vi "Python@SetCaptureFile(Worker)__Parameter.vi"(1 "ParamterIn":string) -> (0 "ParamterOut":string)   [LabVIEW 2020]
uses:
  MainFrame/Global.vi
panel:
  in  "Session":string(combo)
  out "Image":T1(plugin-control)
  in  "Picture":string(combo)
  in  "PythonName":string(combo)
  in  "CamName":string(combo)
  in  "Confirm":bool
  # "Python@SetCaptureFile(worker) $Worker,$Capture,$Picture,$PythonName"
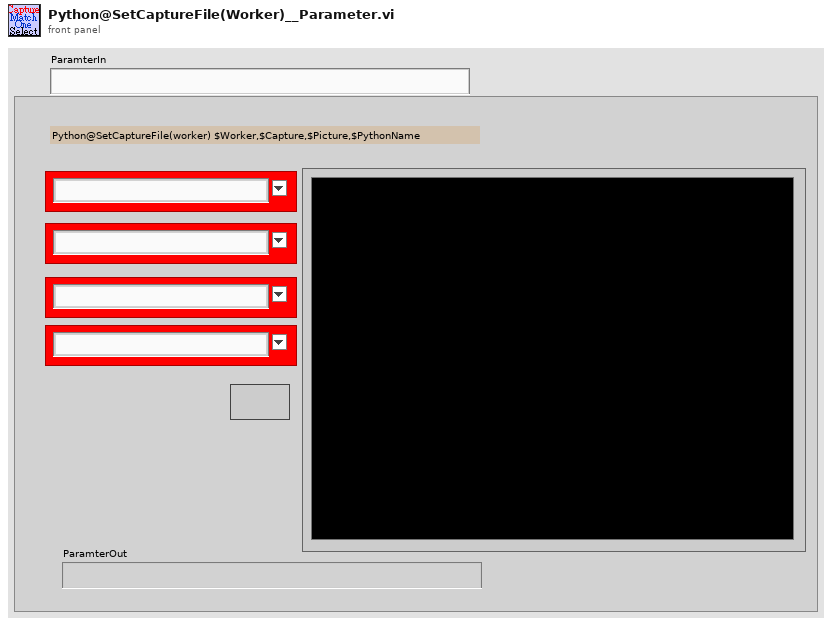
[diagram p1: front panel]
types:
  T1 = typedef "IMAQ Image.ctl" = refnum<image>
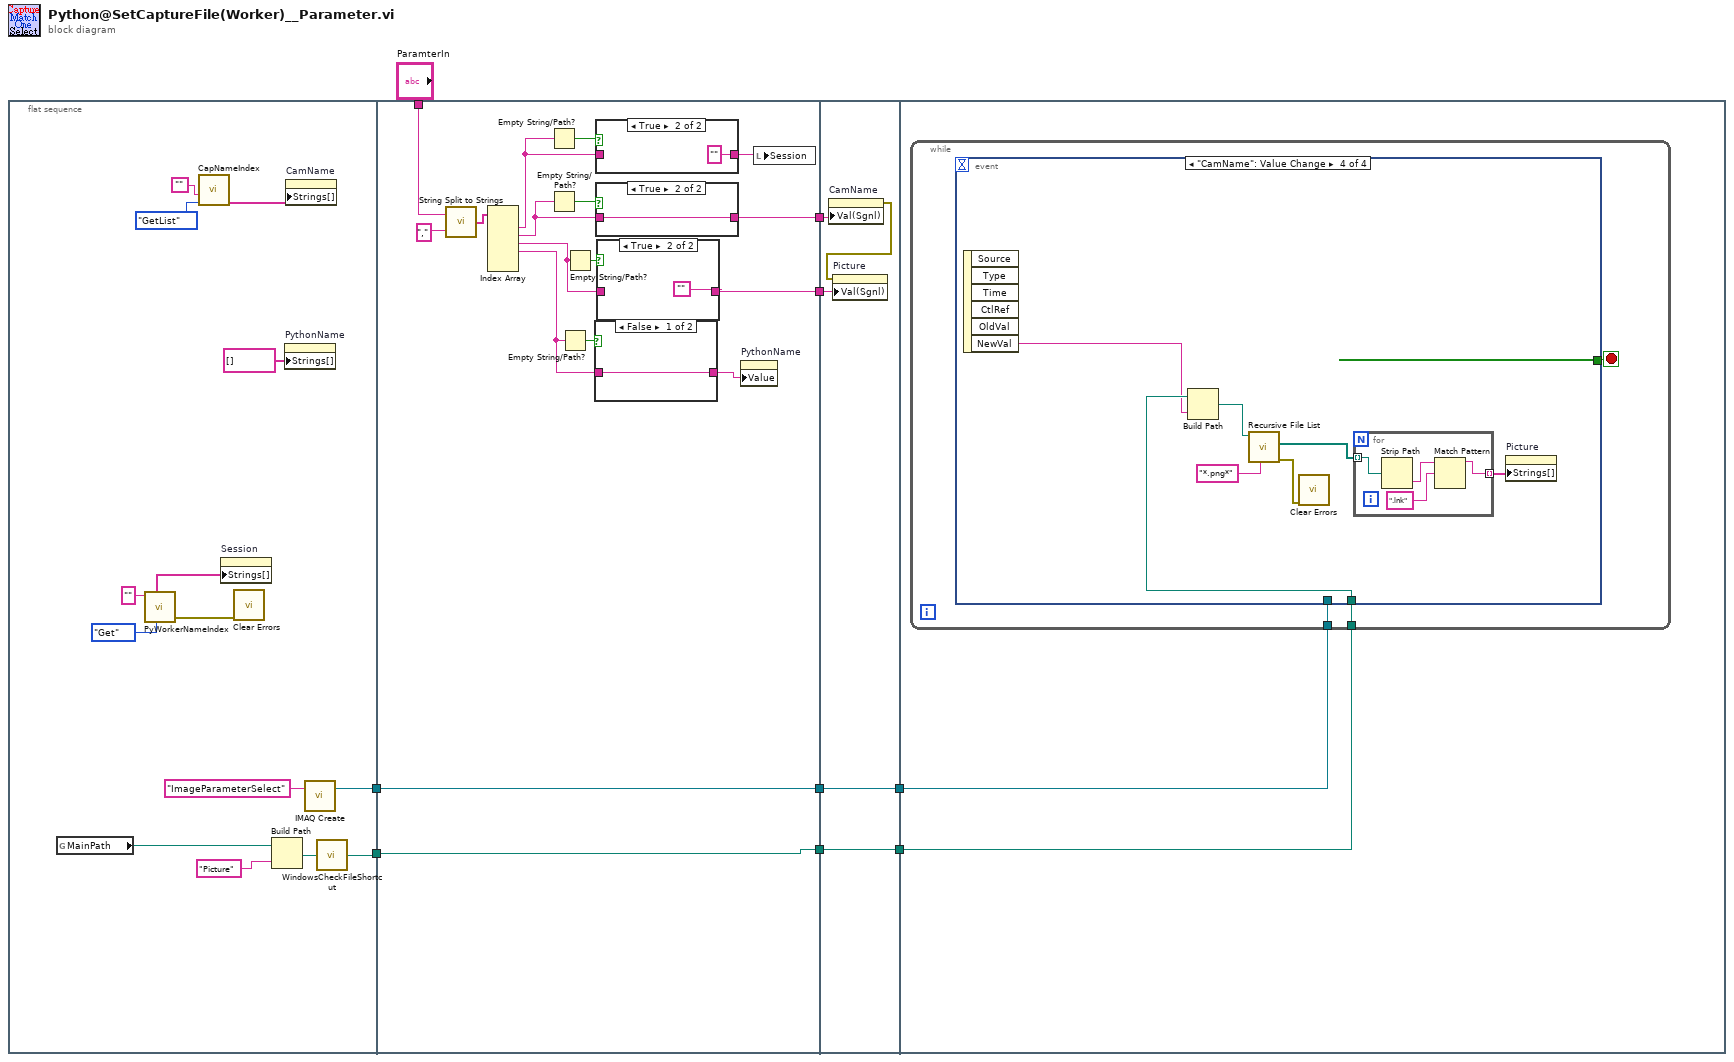
[diagram p0: block diagram]
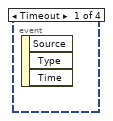
[diagram p6: hidden frame]
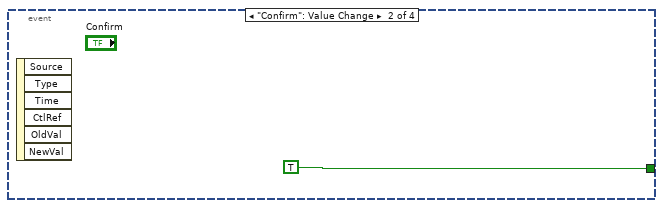
[diagram p7: hidden frame]
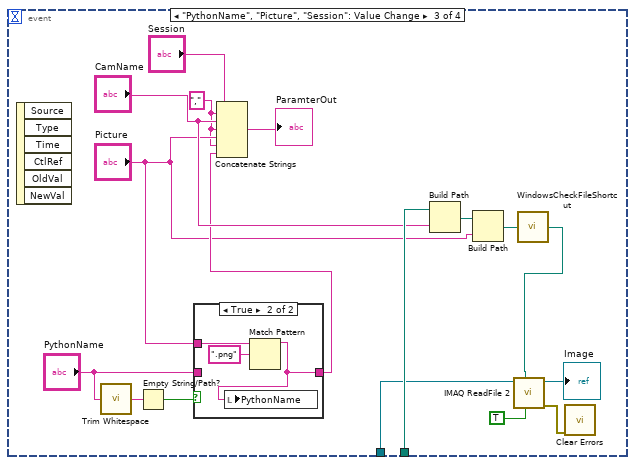
[diagram p8: hidden frame]
diagram:
  n1 = flat-sequence {
    tunnel: [w19] -> w8
    tunnel: [w10] -> w3
    tunnel: "ParamterIn" -> [w38]
    tunnel: w8 -> [w31]
    tunnel: [w31] -> w7
    tunnel: [w29] -> w4
    tunnel: w3 -> [w29]
    tunnel: [w28] -> w2
    tunnel: [w27] -> w1
    tunnel: w7 -> [w53]
    tunnel: [w53] -> w6
    tunnel: [w52] -> w5
    tunnel: w4 -> [w52]
    tunnel: w2 -> [w51]
    tunnel: w1 -> [w49]
    tunnel: w6 -> [w55]
    tunnel: w5 -> [w54]
    frame #0 {
      n2 = global read "Global.vi" "MainPath"() -> (w17:path)
      n3 = call "PyWorkerNameIndex.vi"("OP"=enum16{"Init", "Get", "Set"}."Get", "WrokerName"="" ("SessionIn")) -> ("error out"=w12:errorcluster, "PythonWorkerNameS"=w13:string[])  [unwired: 6 in, 2 out]
      n4 = call "CapNameIndex.vi"("OP"=enum16{"AddCam", "GetIndex", "Init", "GetList"}."GetList", "CamName"="") -> ("DeviceList"=w22:string[])  [unwired: 2 in, 3 out]
      n5 = property on="Session" class="CmbBox"("Strings[]"=w13) -> ()  [unwired: 2 in, 2 out]
      n6 = call <vilib>:"Clear Errors.vi"("error in (no error)"=w12) -> ()  [unwired: 5 in, 2 out]
      n7 = Build Path(base path=w17, name or relative path="Picture") -> (appended path=w11:path)
      n8 = property on="PythonName" class="CmbBox"("Strings[]"=string[] [] ("Strings []")) -> ()  [unwired: 2 in, 2 out]
      n9 = property on="CamName" class="CmbBox"("Strings[]"=w22) -> ()  [unwired: 2 in, 2 out]
      n10 = call "IMAQ Create"("Image Name"="ImageParameterSelect") -> ("New Image"=w19:T1)  [unwired: 4 in, 1 out]
      n11 = call "WindowsCheckFileShortcut.vi"("LinkPath"=w11) -> ("TargetPath"=w10:path)  [unwired: 4 in]
    }
    frame #1 {
      n12 = call "String Split to Strings.vi"("search string/char (-)"=",", "String"=w38) -> ("Array"=w40:string[])
      n13 = Index Array(array=w40) -> (element #1=w25:string, element #2=w30:string, element #3=w32:string, element #4=w35:string)  [unwired: 6 in, 2 out]
      n14 = Empty String/Path?(string/path=w25) -> (empty?=w26:bool)
      n15 = Empty String/Path?(string/path=w30) -> (empty?=w37:bool)
      n16 = Empty String/Path?(string/path=w35) -> (empty?=w36:bool)
      n17 = Empty String/Path?(string/path=w32) -> (empty?=w33:bool)
      n18 = case shown="False" w36 {
        tunnel: [w45 w46] -> w34
        tunnel: w35 -> [w45 w46]
        frame False {
        }
        frame True {
        }
      }
      n19 = case shown="True" w26 {
        tunnel: w25 -> [w41 _]
        tunnel: [w41 ""] -> w24
        frame False {
        }
        frame True {
        }
      }
      n20 = case shown="True" w37 {
        tunnel: w30 -> [w47 w48]
        tunnel: [w47 w48] -> w27
        frame False {
        }
        frame True {
        }
      }
      n21 = case shown="True" w33 {
        tunnel: [w43 ""] -> w28
        tunnel: w32 -> [w43 _]
        frame False {
        }
        frame True {
        }
      }
      n22 = property on="PythonName" class="CmbBox"("Value"=w34) -> ()  [unwired: 2 in, 2 out]
      n23 = local write "Session"(w24) -> ()
    }
    frame #2 {
      n24 = property on="CamName" class="CmbBox"("Val(Sgnl)"=w49) -> (error out=w50:errorcluster)  [unwired: 2 in, 1 out]
      n25 = property on="Picture" class="CmbBox"(error in=w50, "Val(Sgnl)"=w51) -> ()  [unwired: 1 in, 2 out]
    }
    frame #3 {
      n26 = while {
        tunnel: w55 -> [w57]
        tunnel: w54 -> [w56]
        stop <- w58 stop-if-true
        n27 = event shown="[3] \"CamName\": Value Change" {
          selector: _ -> [_ _ _ _]
          dyn-events: _ -> [_ _ _ _]
          timeout: _ -> [_ _ _ _]
          tunnel: [_ TRUE _ _] -> w58
          tunnel: w57 -> [_ _ w65 _]
          tunnel: w56 -> [_ _ w75 w84]
          event Timeout {
            n28 = event-data() -> ()  [unwired: 1 in, 3 out]
          }
          event "Confirm": Value Change {
            n29 = event-data() -> ()  [unwired: 1 in, 6 out]
          }
          event "PythonName", "Picture", "Session": Value Change {
            w63 = "," ("string")
            n30 = event-data() -> ()  [unwired: 1 in, 6 out]
            n31 = call <vilib>:"Trim Whitespace.vi"("string"="PythonName") -> ("trimmed string"=w70:string)  [unwired: 1 in]
            n32 = Empty String/Path?(string/path=w70) -> (empty?=w69:bool)
            n33 = case shown="True" w69 {
              tunnel: "PythonName" -> [w77 _]
              tunnel: [w77 w78] -> w67
              tunnel: "Picture" -> [_ w80]
              frame False {
              }
              frame True {
                n34 = Match Pattern(string=w80, regular expression=".png") -> (before substring=w78:string)  [unwired: 1 in, 3 out]
                n35 = local write "PythonName"(w78) -> ()
              }
            }
            n36 = Concatenate Strings("Session", w63, "CamName", w63, "Picture", w63, w67) -> (→"ParamterOut":string)
            n37 = Build Path(base path=w75, name or relative path="CamName") -> (appended path=w73:path)
            n38 = Build Path(base path=w73, name or relative path="Picture") -> (appended path=w61:path)
            n39 = call "WindowsCheckFileShortcut.vi"("LinkPath"=w61) -> ("TargetPath"=w60:path)  [unwired: 4 in]
            n40 = call "IMAQ ReadFile 2"("Use File Path Image Type"=TRUE, "File Path"=w60, "Image"=w65) -> ("error out"=w72:errorcluster, "Image Out"=→"Image":T1)  [unwired: 4 in, 3 out]
            n41 = call <vilib>:"Clear Errors.vi"("error in (no error)"=w72) -> ()  [unwired: 5 in, 2 out]
          }
          event "CamName": Value Change {
            n42 = event-data() -> ("NewVal"=w83:string)  [unwired: 1 in, 5 out]
            n43 = Build Path(base path=w84, name or relative path=w83) -> (appended path=w82:path)
            n44 = call <vilib>:"Recursive File List.vi"("pattern"="*.png*", "Folder Path"=w82) -> ("error out"=w81:errorcluster, "All Files in Dir"=w86:path[])  [unwired: 5 in, 3 out]
            n45 = call <vilib>:"Clear Errors.vi"("error in (no error)"=w81) -> ()  [unwired: 5 in, 2 out]
            n46 = for {
              tunnel: w86 -> [w91] mode=indexing
              tunnel: [w90] -> w87 mode=indexing
              n47 = Strip Path(path=w91) -> (name=w89:string)  [unwired: 1 out]
              n48 = Match Pattern(string=w89, regular expression=".lnk") -> (before substring=w90:string)  [unwired: 1 in, 3 out]
            }
            n49 = property on="Picture" class="CmbBox"("Strings[]"=w87) -> ()  [unwired: 2 in, 2 out]
          }
        }
      }
    }
  }
